vi "Get Tuning(u32).vi"(7 "section":string, 8 "error in (no error)":errorcluster, 9 "default value":u32, 10 "key":string, 11 "Config File refnum":T1) -> (0 "error out":errorcluster, 1 "value":u32, 3 "Config File refnum out":T1)   [LabVIEW 2014, in "Robot Actor Framework.lvlib" / "Utilities.lvlib"]
uses:
  Utilities.lvlib
  <vilib>/Utility/config.llb/Config Data RefNum.ctl
  <vilib>/Utility/config.llb/Read Key (U32).vi
  <vilib>/Utility/config.llb/Write Key (U32).vi
  <vilib>/Utility/config.llb/NI_LVConfig.lvlib
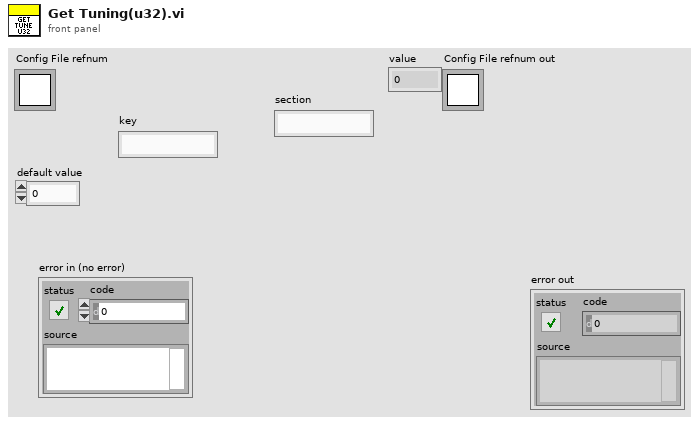
[diagram p1: front panel]
types:
  T1 = typedef "NI_LVConfig.lvlib/Config Data RefNum.ctl" = refnum<k1>
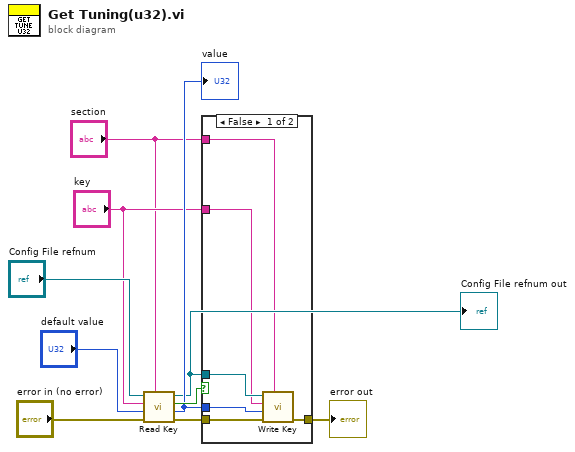
[diagram p0: block diagram]
diagram:
  n1 = call-poly <vilib>:"Read Key.vi"("section"="section", "error in (no error)"="error in (no error)", "default value"="default value", "key"="key", "refnum"="Config File refnum") -> ("error out"=w2:errorcluster, "value"=w7:u32, "found?"=w8:bool, "refnum out"=w6:T1)  [unwired: 3 in]
  "value" <- w7
  "Config File refnum out" <- w6
  n2 = case shown="False" w8 {
    tunnel: w7 -> [w16 _]
    tunnel: w6 -> [w15 _]
    tunnel: "key" -> [w14 _]
    tunnel: "section" -> [w13 _]
    tunnel: w2 -> [w12 w17]
    tunnel: [w11 w17] -> w1
    frame False {
      n3 = call-poly <vilib>:"Write Key.vi"("section"=w13, "error in (no error)"=w12, "value"=w16, "key"=w14, "refnum"=w15) -> ("error out"=w11:errorcluster)  [unwired: 4 in, 2 out]
    }
    frame True {
    }
  }
  "error out" <- w1
